vi "Teleop.vi"(10 "Match Info":T2={"Autonomous Elapsed Seconds"=0.0, "TeleOp Elapsed Seconds"=0.0, "Disabled Elapsed Seconds"=0.0, "Visited Autonomous"=FALSE, "Visited TeleOp"=FALSE, "Visited Disabled"=FALSE, "Autonomous Settings"={"Autonomous Style"=enum."Independent", "VI Refnum"=refnum}}, 11 "Call Context":T3=enum."Execute") -> ()   [LabVIEW 2018]
doc: "This VI is called for each TeleOp packet received from the DS where the robot is not disabled. It is often used to read from the joysticks and update I/O or to update setpoints for timed control loops. It should complete and return within 20 milliseconds or it may miss DS packets."
uses:
  <vilib>/Rock Robotics/WPI/DriverStation/WPI_DriverStationDerivedRobotMode.ctl
  <vilib>/Rock Robotics/WPI/DriverStation/WPI_DriverStationMatch Info.ctl
  <vilib>/Rock Robotics/WPI/Utilities/WPI_GetSetVariantRefNum.vi
  <vilib>/Rock Robotics/Network Tables/NT Write Boolean Array.vi
  <vilib>/Rock Robotics/Network Tables/NT Write Numeric Array.vi
  <vilib>/Rock Robotics/Network Tables/NT Read Boolean.vi
  <vilib>/Rock Robotics/Network Tables/NT Read Number.vi
  <vilib>/Rock Robotics/WPI/RobotDrive/WPI_RobotDriveArcadeDrive_Standard(NoSaturation).vi
  Robot Global Data.vi
  <vilib>/addons/control/pid/NI_PID_pid.lvlib
  <vilib>/Rock Robotics/WPI/ThirdParty/Phoenix-LabVIEW/Motor Controller/Controls/CTRE_Phoenix_MotorControl_ControlMode.ctl
  <vilib>/addons/control/pid/pid.llb/PID (DBL).vi
  <vilib>/Rock Robotics/WPI/ThirdParty/Phoenix-LabVIEW/Motor Controller/Get/CTRE_Phoenix_MotorController_GetQuadratureData.vi
  <vilib>/Rock Robotics/Network Tables/NT Write Boolean.vi
panel:
  in  "Sync PID":T1={"proportional gain (Kc)"=1.0, "integral time (Ti, min)"=0.01, "derivative time (Td, min)"=0.0} {"derivative time (Td, min)" format="%.3f"; "integral time (Ti, min)" format="%.3f"; "proportional gain (Kc)" format="%.3f"}
  in  "Drive PID":T1={"proportional gain (Kc)"=1.0, "integral time (Ti, min)"=0.01, "derivative time (Td, min)"=0.0} {"derivative time (Td, min)" format="%.3f"; "integral time (Ti, min)" format="%.3f"; "proportional gain (Kc)" format="%.3f"}
  in  "Mode":string(combo)="Driving"
  out "Drive Type":bool
  out "Sample Slider 0":dbl(slide) scale=0.0..5.0
  out "Sample Boolean 1":bool
  out "Sample Boolean 0":bool
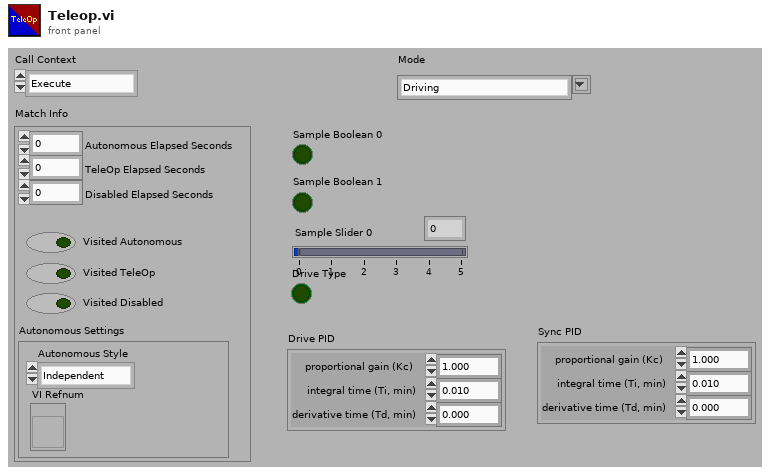
[diagram p1: front panel]
types:
  T1 = cluster{"proportional gain (Kc)":dbl, "integral time (Ti, min)":dbl, "derivative time (Td, min)":dbl}
  T2 = typedef "WPI_DriverStationMatch Info.ctl" = cluster{"Autonomous Elapsed Seconds":dbl, "TeleOp Elapsed Seconds":dbl, "Disabled Elapsed Seconds":dbl, "Visited Autonomous":bool, "Visited TeleOp":bool, "Visited Disabled":bool, "Autonomous Settings":cluster{"Autonomous Style":enum16{"Iterative", "Independent"}, "VI Refnum":refnum<vi>}}
  T3 = typedef "WPI_DriverStationDerivedRobotMode.ctl" = enum16{"Init", "Execute", "Stop"}
  T4 = typedef "WPI_JoystickDevRef.ctl" = cluster{"Device":T5}
  T5 = typedef "WPI_JoystickDeviceEnum.ctl" = enum16{"USB 0", "USB 1", "USB 2", "USB 3", "USB 4", "USB 5"}
  T6 = typedef "CTRE_Phoenix_MotorControl_ControlMode.ctl" = u16
  T7 = cluster{"Yaw":dbl, "Roll":dbl, "Pitch":dbl, "Heading":dbl, "Fused Heading":dbl}
  T8 = typedef "WPI_MotorControlDeviceRef.ctl" = cluster{"DeviceStatus":errorcluster, "Type":T9, "PWM":cluster{"PWM Channel":T10, "DeadBand":T11}, "CAN":cluster{"Device Number":u8, "SetOutput VI Ref":variant, "GetOutput VI Ref":variant, "Enable VI Ref":variant, "Disable VI Ref":variant, "Data":variant}, "Invert":bool, "DIO PWM":cluster{"PWM \"Enable\" Channel":T10, "DIOChannel":T12, "PWM Rate":dbl}}
  T9 = typedef "WPI_MotorControlType.ctl" = enum16{"PWM", "CAN", "DIO PWM"}
  T10 = typedef "FPGA_DIOPWMChannel.ctl" = enum8{"PWM 0", "PWM 1", "PWM 2", "PWM 3", "PWM 4", "PWM 5", "PWM 6", "PWM 7", "PWM 8", "PWM 9", "PWM MXP 0", "PWM MXP 1", "PWM MXP 2", "PWM MXP 3", "PWM MXP 4", "PWM MXP 5", "PWM MXP 6", "PWM MXP 7", "PWM MXP 8", "PWM MXP 9", "Invalid"}
  T11 = typedef "WPI_PWMDeadband.ctl" = cluster{"Name":string, "maxPositivePwm":i32, "minPositivePwm":i32, "centerPwm":i32, "maxNegativePwm":i32, "minNegativePwm":i32, "angularRange":u16}
  T12 = typedef "FPGA_DIOChannel.ctl" = enum8{"DIO 0", "DIO 1", "DIO 2", "DIO 3", "DIO 4", "DIO 5", "DIO 6", "DIO 7", "DIO 8", "DIO 9", "DIO MXP 0", "DIO MXP 1", "DIO MXP 2", "DIO MXP 3", "DIO MXP 4", "DIO MXP 5", "DIO MXP 6", "DIO MXP 7", "DIO MXP 8", "DIO MXP 9", "DIO MXP 10", "DIO MXP 11", "DIO MXP 12", "DIO MXP 13", "DIO MXP 14", "DIO MXP 15", "SPI Port CS1", "SPI Port CS2", "SPI Port CS3", "SPI Port MISO", "SPI Port MOSI", "Invalid"}
  T13 = typedef "WPI_RobotDriveDevRef.ctl" = cluster{"DevStatus":errorcluster, "Motors[]":T8[], "Square Inputs":bool, "Max Output":dbl}
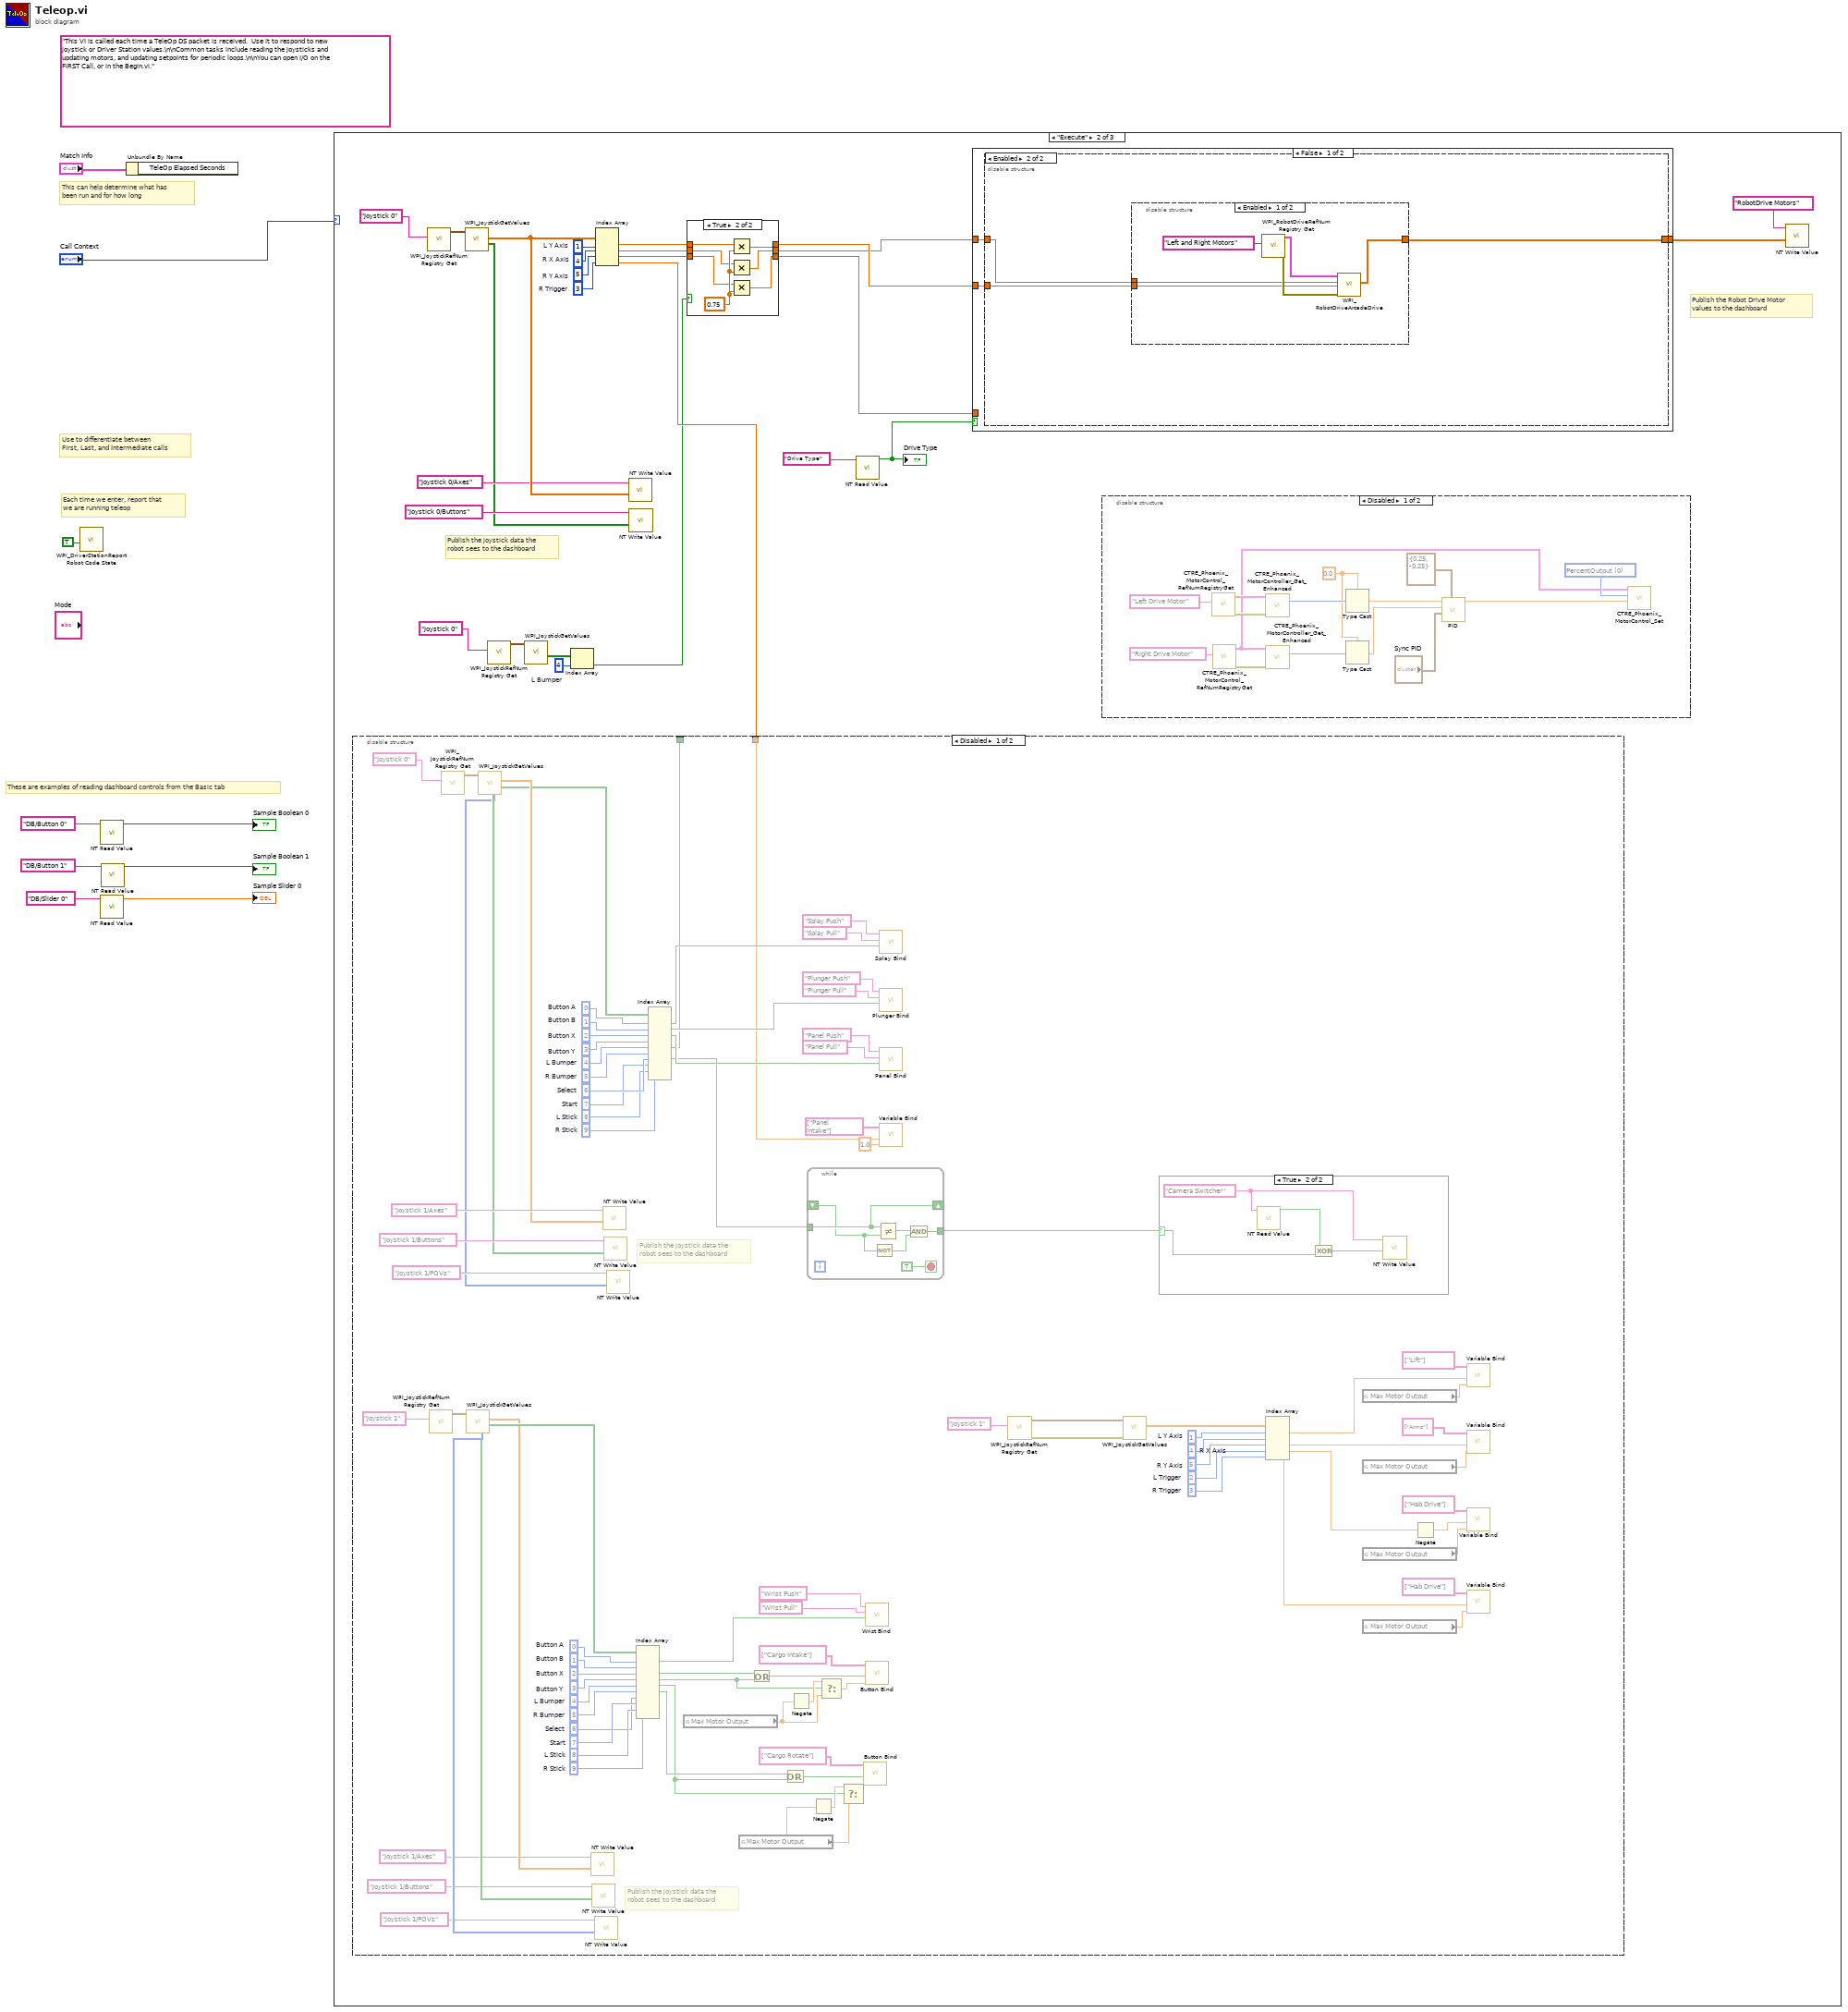
[diagram p0: block diagram]
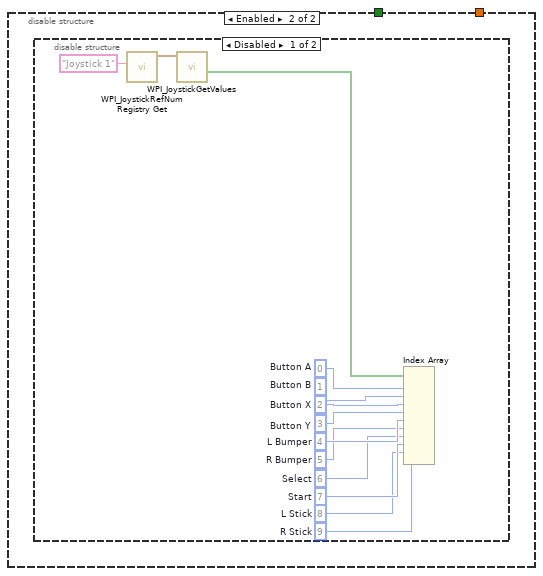
[diagram p4: hidden frame]
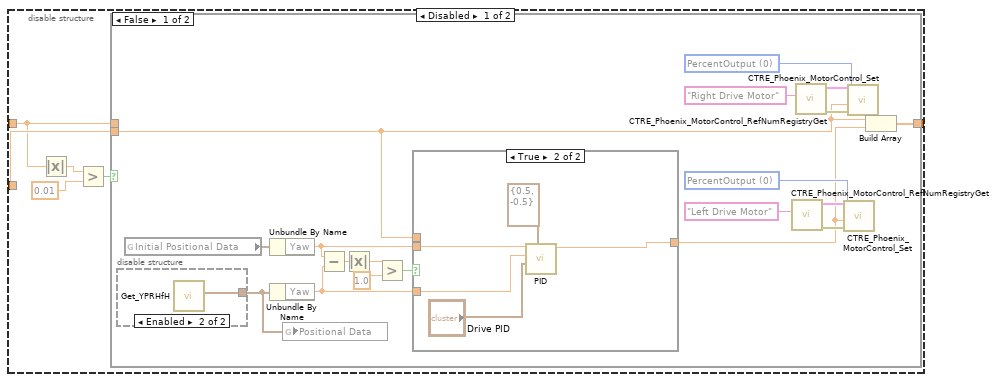
[diagram p7: hidden frame]
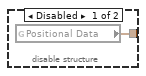
[diagram p8: hidden frame]
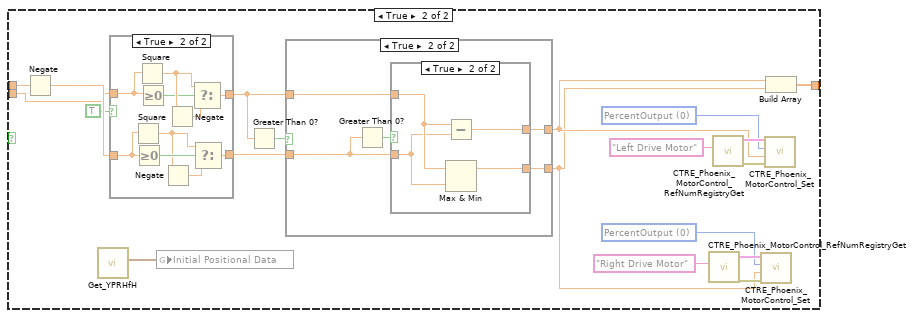
[diagram p10: hidden frame]
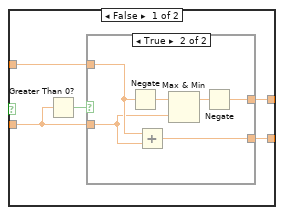
[diagram p11: hidden frame]
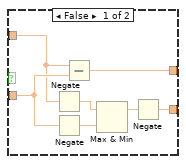
[diagram p12: hidden frame]
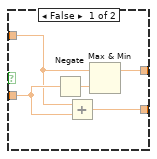
[diagram p13: hidden frame]
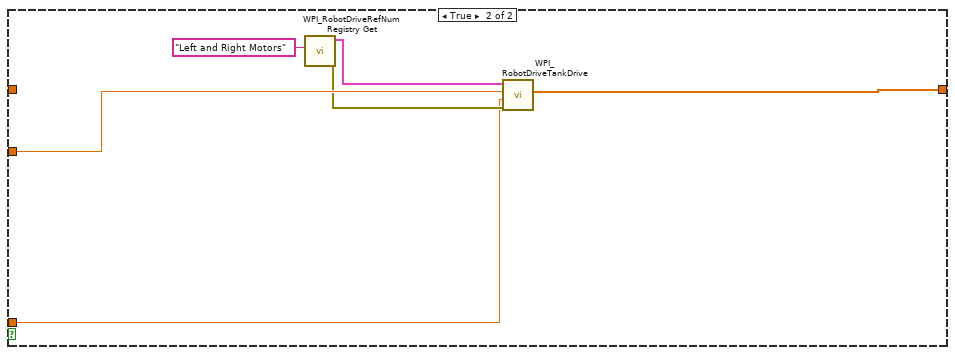
[diagram p16: hidden frame]
diagram:
  (unwired) "This VI is called each time a TeleOp DS packet is received.  Use it to respond to new joystick or Driver Station values.\n\nCommon tasks include reading the joysticks and updating motors, and updating setpoints for periodic loops.\n\nYou can open I/O on the FIRST Call, or in the Begin.vi."
  # "These are examples of reading dashboard controls from the Basic tab"
  # "Each time we enter, report that\nwe are running teleop"
  # "Use to differentiate between\nFirst, Last, and Intermediate calls"
  # "This can help determine what has\nbeen run and for how long"
  n1 = call <vilib>:"WPI_DriverStationReport Robot Code State.vi"("TeleOp"=TRUE ("Autonomous")) -> ()  [unwired: 10 in, 1 out]
  n2 = call-poly <vilib>:"NT Read Value.vi"("Name"="DB/Button 0" ("refnum name")) -> ("Boolean"=→"Sample Boolean 0":bool)  [unwired: 9 in, 1 out]
  n3 = call-poly <vilib>:"NT Read Value.vi"("Name"="DB/Slider 0" ("refnum name")) -> ("Numeric"=→"Sample Slider 0":dbl)  [unwired: 9 in, 1 out]
  n4 = call-poly <vilib>:"NT Read Value.vi"("Name"="DB/Button 1" ("refnum name")) -> ("Boolean"=→"Sample Boolean 1":bool)  [unwired: 9 in, 1 out]
  n5 = Unbundle By Name("Match Info") -> ()  [unwired: 1 out]
  n6 = case shown="\"Execute\"" "Call Context" {
    frame "Init", Default {
    }
    frame "Execute" {
      w12 = 4  # L Bumper
      w17 = 3  # R Trigger
      w28 = 4  # R X Axis
      w29 = 1  # L Y Axis
      w27 = 5  # R Y Axis
      # "Publish the Robot Drive Motor\nvalues to the dashboard"
      # "Publish the joystick data the\nrobot sees to the dashboard"
      n7 = call <vilib>:"WPI_JoystickRefNum Registry Get.vi"("refnum name"="Joystick 0") -> ("JoystickDevRef"=w34:T4)  [unwired: 1 in, 9 out]
      n8 = call <vilib>:"WPI_JoystickGetValues.vi"("JoystickDevRef"=w34) -> ("Buttons"=w26:bool[], "Axes"=w35:dbl[])  [unwired: 6 in, 3 out]
      n9 = call <vilib>:"WPI_JoystickRefNum Registry Get.vi"("refnum name"="Joystick 0") -> ("JoystickDevRef"=w14:T4)  [unwired: 1 in, 9 out]
      n10 = call <vilib>:"WPI_JoystickGetValues.vi"("JoystickDevRef"=w14) -> ("Buttons"=w10:bool[])  [unwired: 6 in, 4 out]
      n11 = Index Array(array=w10, index=w12) -> (element=w11:bool)
      n12 = Index Array(array=w35, index #1=w29, index #2=w28, index #3=w27, index #4=w17) -> (element #1=w25:dbl, element #2=w22:dbl, element #3=w21:dbl, element #4=w16:dbl)
      n13 = disable-structure shown="Disabled" {
        disable-tunnel: [w102 _] -> _
        disable-tunnel: w16 -> [w44 _]
        frame Disabled {
          w60 = 3  # R Trigger
          w61 = 2  # L Trigger
          w63 = 4  # R X Axis
          w64 = 1  # L Y Axis
          w62 = 5  # R Y Axis
          w99 = 9  # R Stick
          w98 = 8  # L Stick
          w97 = 7  # Start
          w96 = 6  # Select
          w95 = 5  # R Bumper
          w94 = 4  # L Bumper
          w82 = 3  # Button Y
          w85 = 1  # Button B
          w83 = 0  # Button A
          w84 = 2  # Button X
          w104 = 9  # R Stick
          w105 = 8  # L Stick
          w106 = 7  # Start
          w107 = 6  # Select
          w112 = 5  # R Bumper
          w113 = 4  # L Bumper
          w125 = 3  # Button Y
          w122 = 1  # Button B
          w124 = 0  # Button A
          w123 = 2  # Button X
          # "Publish the joystick data the\nrobot sees to the dashboard"
          # "Publish the joystick data the\nrobot sees to the dashboard"
          n14 = call <vilib>:"WPI_JoystickRefNum Registry Get.vi"("refnum name"="Joystick 1") -> ("JoystickDevRef"=w87:T4)  [unwired: 1 in, 9 out]
          n15 = call <vilib>:"WPI_JoystickRefNum Registry Get.vi"("refnum name"="Joystick 0") -> ("JoystickDevRef"=w120:T4)  [unwired: 1 in, 9 out]
          n16 = call <vilib>:"WPI_JoystickGetValues.vi"("JoystickDevRef"=w87) -> ("Buttons"=w91:bool[], "Axes"=w90:dbl[], "POVs"=w93:i16[])  [unwired: 6 in, 2 out]
          n17 = call <vilib>:"WPI_JoystickGetValues.vi"("JoystickDevRef"=w120) -> ("Buttons"=w116:bool[], "Axes"=w117:dbl[], "POVs"=w114:i16[])  [unwired: 6 in, 2 out]
          n18 = call-poly <vilib>:"NT Write Value.vi"("Numeric Array"=w90, "Name"="Joystick 1/Axes") -> ()  [unwired: 9 in, 1 out]
          n19 = call-poly <vilib>:"NT Write Value.vi"("Boolean Array"=w91, "Name"="Joystick 1/Buttons") -> ()  [unwired: 9 in, 1 out]
          n20 = call-poly <vilib>:"NT Write Value.vi"("Numeric Array"=w93, "Name"="Joystick 1/POVs") -> ()  [unwired: 9 in, 1 out]
          n21 = call-poly <vilib>:"NT Write Value.vi"("Numeric Array"=w117, "Name"="Joystick 1/Axes") -> ()  [unwired: 9 in, 1 out]
          n22 = call-poly <vilib>:"NT Write Value.vi"("Boolean Array"=w116, "Name"="Joystick 1/Buttons") -> ()  [unwired: 9 in, 1 out]
          n23 = call-poly <vilib>:"NT Write Value.vi"("Numeric Array"=w114, "Name"="Joystick 1/POVs") -> ()  [unwired: 9 in, 1 out]
          n24 = Index Array(array=w91, index #1=w83, index #2=w85, index #3=w84, index #4=w82, index #5=w94, index #6=w95, index #7=w96, index #8=w97, index #9=w98, index #10=w99) -> (element #1=w77:bool, element #3=w40:bool, element #4=w37:bool, element #5=w36:bool, element #6=w81:bool)  [unwired: 5 out]
          n25 = Index Array(array=w116, index #1=w124, index #2=w122, index #3=w123, index #4=w125, index #5=w113, index #6=w112, index #7=w107, index #8=w106, index #9=w105, index #10=w104) -> (element #1=w108:bool, element #2=w111:bool, element #3=w103:bool, element #5=w102:bool, element #7=w46:bool)  [unwired: 5 out]
          n26 = global read "Robot Global Data.vi" "Max Motor Output"() -> (w41:dbl)
          n27 = global read "Robot Global Data.vi" "Max Motor Output"() -> (w73:dbl)
          n28 = Or(x=w40, y=w37) -> (x .or. y?=w38:bool)
          n29 = Or(x=w81, y=w36) -> (x .or. y?=w76:bool)
          n30 = Negate(x=w41) -> (-x=w42:dbl)
          n31 = while {
            shift-right: [w135] -> _
            shift-left: _ -> [w133]
            tunnel: w46 -> [w135]
            tunnel: [w132] -> w45
            stop <- TRUE stop-if-true
            n32 = Not(x=w133) -> (.not. x?=w130:bool)
            n33 = Not Equal?(x=w135, y=w133) -> (x != y?=w131:bool)
            n34 = And(x=w131, y=w130) -> (x .and. y?=w132:bool)
          }
          n35 = Negate(x=w73) -> (-x=w74:dbl)
          n36 = Select(t=w42, s=w37, f=w41) -> (s? t:f=w39:dbl)
          n37 = Select(t=w74, s=w36, f=w73) -> (s? t:f=w75:dbl)
          n38 = call "Button Bind.vi"("Output"=w75, "Button ID"=w76, "PhoenixMotorControlDevRef"=string[] ["Cargo Rotate"] ("Motor Controllers")) -> ()  [unwired: 8 in, 1 out]
          n39 = call "Wrist Bind.vi"("Button Input"=w77, "Pull Solenoid Ref"="Wrist Pull" ("Push Solenoid Ref"), "Push Solenoid Ref"="Wrist Push") -> ()  [unwired: 9 in]
          n40 = call "Button Bind.vi"("Output"=w39, "Button ID"=w38, "PhoenixMotorControlDevRef"=string[] ["Cargo Intake"] ("Motor Controllers")) -> ()  [unwired: 8 in, 1 out]
          n41 = call "Splay Bind.vi"("Button Input"=w108, "Pull Solenoid Ref"="Splay Pull" ("Push Solenoid Ref"), "Push Solenoid Ref"="Splay Push") -> ()  [unwired: 9 in]
          n42 = call "Plunger Bind.vi"("Button Input"=w111, "Pull Solenoid Ref"="Plunger Pull" ("Push Solenoid Ref"), "Push Solenoid Ref"="Plunger Push") -> ()  [unwired: 9 in]
          n43 = call "Panel Bind.vi"("Button Input"=w103, "Pull Solenoid Ref"="Panel Pull" ("Push Solenoid Ref"), "Push Solenoid Ref"="Panel Push") -> ()  [unwired: 9 in]
          n44 = call "Variable Bind.vi"("Ouput"=1.0 ("Max Ouput"), "Axis ID"=w44, "PhoenixMotorControlDevRef"=string[] ["Panel Intake"] ("Motor Controllers")) -> ()  [unwired: 8 in, 1 out]
          n45 = call <vilib>:"WPI_JoystickRefNum Registry Get.vi"("refnum name"="Joystick 1") -> ("error out"=w66:errorcluster, "JoystickDevRef"=w67:T4)  [unwired: 1 in, 8 out]
          n46 = call <vilib>:"WPI_JoystickGetValues.vi"("error in (no error)"=w66, "JoystickDevRef"=w67) -> ("Axes"=w65:dbl[])  [unwired: 5 in, 4 out]
          n47 = case shown="True" w45 {
            selector: w45 -> [_ w129]
            frame False {
            }
            frame True {
              w127 = "Camera Switcher" ("Name")
              n48 = call-poly <vilib>:"NT Read Value.vi"("Name"=w127) -> ("Boolean"=w126:bool)  [unwired: 9 in, 1 out]
              n49 = Exclusive Or(1:w129, 2:w126) -> (0:w128:bool)
              n50 = call-poly <vilib>:"NT Write Value.vi"("Boolean"=w128, "Name"=w127) -> ()  [unwired: 9 in, 1 out]
            }
          }
          n51 = Index Array(array=w65, index #1=w64, index #2=w63, index #3=w62, index #4=w61, index #5=w60) -> (element #1=w50:dbl, element #3=w49:dbl, element #4=w58:dbl, element #5=w53:dbl)  [unwired: 1 out]
          n52 = global read "Robot Global Data.vi" "Max Motor Output"() -> (w51:dbl)
          n53 = global read "Robot Global Data.vi" "Max Motor Output"() -> (w47:dbl)
          n54 = global read "Robot Global Data.vi" "Max Motor Output"() -> (w56:dbl)
          n55 = global read "Robot Global Data.vi" "Max Motor Output"() -> (w55:dbl)
          n56 = Negate(x=w58) -> (-x=w57:dbl)
          n57 = call "Variable Bind.vi"("Ouput"=w51, "Axis ID"=w50, "PhoenixMotorControlDevRef"=string[] ["Lift"] ("Motor Controllers")) -> ()  [unwired: 8 in, 1 out]
          n58 = call "Variable Bind.vi"("Ouput"=w47, "Axis ID"=w49, "PhoenixMotorControlDevRef"=string[] ["Arms"] ("Motor Controllers")) -> ()  [unwired: 8 in, 1 out]
          n59 = call "Variable Bind.vi"("Ouput"=w56, "Axis ID"=w57, "PhoenixMotorControlDevRef"=string[] ["Hab Drive"] ("Motor Controllers")) -> ()  [unwired: 8 in, 1 out]
          n60 = call "Variable Bind.vi"("Ouput"=w55, "Axis ID"=w53, "PhoenixMotorControlDevRef"=string[] ["Hab Drive"] ("Motor Controllers")) -> ()  [unwired: 8 in, 1 out]
        }
        frame Enabled {
          n61 = disable-structure shown="Disabled" {
            frame Disabled {
              w138 = 9  # R Stick
              w139 = 8  # L Stick
              w140 = 7  # Start
              w141 = 6  # Select
              w142 = 5  # R Bumper
              w143 = 4  # L Bumper
              w144 = 3  # Button Y
              w146 = 1  # Button B
              w147 = 0  # Button A
              w145 = 2  # Button X
              n62 = call <vilib>:"WPI_JoystickRefNum Registry Get.vi"("refnum name"="Joystick 1") -> ("JoystickDevRef"=w148:T4)  [unwired: 1 in, 9 out]
              n63 = call <vilib>:"WPI_JoystickGetValues.vi"("JoystickDevRef"=w148) -> ("Buttons"=w137:bool[])  [unwired: 6 in, 4 out]
              n64 = Index Array(array=w137, index #1=w147, index #2=w146, index #3=w145, index #4=w144, index #5=w143, index #6=w142, index #7=w141, index #8=w140, index #9=w139, index #10=w138) -> ()  [unwired: 10 out]
            }
            frame Enabled {
            }
          }
        }
      }
      n65 = call-poly <vilib>:"NT Write Value.vi"("Numeric Array"=w35, "Name"="Joystick 0/Axes") -> ()  [unwired: 9 in, 1 out]
      n66 = call-poly <vilib>:"NT Write Value.vi"("Boolean Array"=w26, "Name"="Joystick 0/Buttons") -> ()  [unwired: 9 in, 1 out]
      n67 = case shown="True" w11 {
        tunnel: w25 -> [w280 w286]
        tunnel: [w280 w285] -> w24
        tunnel: [w279 w283] -> w23
        tunnel: w22 -> [w279 w284]
        tunnel: [w278 w281] -> w20
        tunnel: w21 -> [w278 w282]
        frame False {
        }
        frame True {
          w287 = 0.75 ("y")
          n68 = Multiply(x=w286, y=w287) -> (x*y=w285:dbl)
          n69 = Multiply(x=w284, y=w287) -> (x*y=w283:dbl)
          n70 = Multiply(x=w282, y=w287) -> (x*y=w281:dbl)
        }
      }
      n71 = call-poly <vilib>:"NT Read Value.vi"("Name"="Drive Type" ("refnum name")) -> ("Boolean"=w18:bool)  [unwired: 9 in, 1 out]
      "Drive Type" <- w18
      n72 = case shown="False" w18 {
        tunnel: w20 -> [_ w272]
        tunnel: w23 -> [w165 _]
        tunnel: w24 -> [w166 w277]
        tunnel: [w164 w273] -> w15
        frame False {
          n73 = disable-structure shown="Enabled" {
            disable-tunnel: w166 -> [w172 w264]
            disable-tunnel: w165 -> [w167 w265]
            disable-tunnel: [w168 w263] -> w164
            frame Disabled {
              n74 = Absolute Value(x=w167) -> (abs(x)=w170:dbl)
              n75 = Greater?(x=w170, y=0.01) -> (0:w169:bool)
              n76 = case shown="False" w169 {
                tunnel: [w182 w211] -> w168
                tunnel: w172 -> [w176 w213]
                tunnel: w167 -> [_ w218]
                frame False {
                  w187 = T6 0 items=["PercentOutput"=0, "Position"=1, "Velocity"=2, "Current"=3, "Follower"=5, "MotionProfile"=6, "MotionMagic"=7, "MotionProfileArc"=10, "Disabled"=15] ("Control Mode")
                  w188 = T6 0 items=["PercentOutput"=0, "Position"=1, "Velocity"=2, "Current"=3, "Follower"=5, "MotionProfile"=6, "MotionMagic"=7, "MotionProfileArc"=10, "Disabled"=15] ("Control Mode")
                  n77 = disable-structure shown="Enabled" {
                    disable-tunnel: [w192 w193] -> w173
                    frame Disabled {
                      n78 = global read "Robot Global Data.vi" "Positional Data"() -> (w192:T7)
                    }
                    frame Enabled {
                      n79 = call <vilib>:"Get_YPRHfH.vi"() -> ("YRPHfH"=w193:T7)  [unwired: 11 in]
                    }
                  }
                  n80 = global read "Robot Global Data.vi" "Initial Positional Data"() -> (w181:T7)
                  n81 = Unbundle By Name(w181) -> ("Yaw"=w179:dbl)
                  n82 = Unbundle By Name(w173) -> ("Yaw"=w175:dbl)
                  n83 = global write "Robot Global Data.vi" "Positional Data"(w173) -> ()
                  n84 = Subtract(x=w179, y=w175) -> (x-y=w180:dbl)
                  n85 = Absolute Value(x=w180) -> (abs(x)=w177:dbl)
                  n86 = Greater?(x=w177, y=1.0) -> (0:w174:bool)
                  n87 = case shown="True" w174 {
                    tunnel: w175 -> [_ w199]
                    tunnel: [w194 w196] -> w183
                    tunnel: w176 -> [w194 _]
                    tunnel: w179 -> [_ w197]
                    frame False {
                    }
                    frame True {
                      n88 = call-poly <vilib>:"PID.vi"("output range"=cluster{"output high":dbl, "output low":dbl} {"output high"=0.5, "output low"=-0.5}, "PID gains"="Drive PID", "process variable"=w199, "setpoint"=w197) -> ("output"=w196:dbl)  [unwired: 6 in, 1 out]
                    }
                  }
                  n89 = call <vilib>:"CTRE_Phoenix_MotorControl_RefNumRegistryGet.vi"("refnum name"="Left Drive Motor") -> ("error out"=w185:errorcluster, "PhoenixMotorControlDevRef"=w186:T8)  [unwired: 9 in]
                  n90 = call <vilib>:"CTRE_Phoenix_MotorControl_RefNumRegistryGet.vi"("refnum name"="Right Drive Motor") -> ("error out"=w190:errorcluster, "PhoenixMotorControlDevRef"=w189:T8)  [unwired: 9 in]
                  n91 = call <vilib>:"CTRE_Phoenix_MotorControl_Set.vi"("error in (no error)"=w185, "Output"=w183, "Control Mode"=w187, "PhoenixMotorControlDevRef"=w186) -> ()  [unwired: 6 in, 2 out]
                  n92 = call <vilib>:"CTRE_Phoenix_MotorControl_Set.vi"("error in (no error)"=w190, "Output"=w176, "Control Mode"=w188, "PhoenixMotorControlDevRef"=w189) -> ()  [unwired: 6 in, 2 out]
                  n93 = Build Array(w176, w183) -> (w182:dbl[])
                }
                frame True {
                  w206 = T6 0 items=["PercentOutput"=0, "Position"=1, "Velocity"=2, "Current"=3, "Follower"=5, "MotionProfile"=6, "MotionMagic"=7, "MotionProfileArc"=10, "Disabled"=15] ("Control Mode")
                  w204 = T6 0 items=["PercentOutput"=0, "Position"=1, "Velocity"=2, "Current"=3, "Follower"=5, "MotionProfile"=6, "MotionMagic"=7, "MotionProfileArc"=10, "Disabled"=15] ("Control Mode")
                  n94 = Negate(x=w218) -> (-x=w214:dbl)
                  n95 = call <vilib>:"Get_YPRHfH.vi"() -> ("YRPHfH"=w200:T7)  [unwired: 11 in]
                  n96 = case shown="True" TRUE {
                    tunnel: [w251 w262] -> w215
                    tunnel: [w252 w261] -> w216
                    tunnel: w214 -> [w251 w260]
                    tunnel: w213 -> [w252 w259]
                    frame False {
                    }
                    frame True {
                      n97 = Square(x=w260) -> (x^2=w257:dbl)
                      n98 = Greater Or Equal To 0?(x=w260) -> (x >= 0?=w258:bool)
                      n99 = Square(x=w259) -> (x^2=w254:dbl)
                      n100 = Greater Or Equal To 0?(x=w259) -> (x >= 0?=w253:bool)
                      n101 = Negate(x=w257) -> (-x=w256:dbl)
                      n102 = Negate(x=w254) -> (-x=w255:dbl)
                      n103 = Select(t=w254, s=w253, f=w255) -> (s? t:f=w261:dbl)
                      n104 = Select(t=w257, s=w258, f=w256) -> (s? t:f=w262:dbl)
                    }
                  }
                  n105 = global write "Robot Global Data.vi" "Initial Positional Data"(w200) -> ()
                  n106 = Greater Than 0?(x=w216) -> (x > 0?=w217:bool)
                  n107 = case shown="True" w217 {
                    tunnel: w215 -> [w222 w240]
                    tunnel: w216 -> [w221 w239]
                    tunnel: [w220 w238] -> w202
                    tunnel: [w219 w237] -> w201
                    frame False {
                      n108 = Greater Than 0?(x=w222) -> (x > 0?=w223:bool)
                      n109 = case shown="True" w223 {
                        tunnel: w222 -> [w230 w232]
                        tunnel: w221 -> [w228 w233]
                        tunnel: [w224 w234] -> w220
                        tunnel: [w225 w231] -> w219
                        frame False {
                          n110 = Negate(x=w228) -> (-x=w229:dbl)
                          n111 = Negate(x=w230) -> (-x=w227:dbl)
                          n112 = Subtract(x=w228, y=w230) -> (x-y=w224:dbl)
                          n113 = Max & Min(x=w229, y=w227) -> (max(x,y)=w226:dbl)  [unwired: 1 out]
                          n114 = Negate(x=w226) -> (-x=w225:dbl)
                        }
                        frame True {
                          n115 = Negate(x=w233) -> (-x=w236:dbl)
                          n116 = Add(x=w233, y=w232) -> (x+y=w231:dbl)
                          n117 = Max & Min(x=w236, y=w232) -> (max(x,y)=w235:dbl)  [unwired: 1 out]
                          n118 = Negate(x=w235) -> (-x=w234:dbl)
                        }
                      }
                    }
                    frame True {
                      n119 = Greater Than 0?(x=w240) -> (x > 0?=w241:bool)
                      n120 = case shown="True" w241 {
                        tunnel: w240 -> [w246 w248]
                        tunnel: w239 -> [w243 w249]
                        tunnel: [w244 w247] -> w238
                        tunnel: [w242 w250] -> w237
                        frame False {
                          n121 = Negate(x=w246) -> (-x=w245:dbl)
                          n122 = Add(x=w243, y=w246) -> (x+y=w242:dbl)
                          n123 = Max & Min(x=w243, y=w245) -> (max(x,y)=w244:dbl)  [unwired: 1 out]
                        }
                        frame True {
                          n124 = Subtract(x=w249, y=w248) -> (x-y=w247:dbl)
                          n125 = Max & Min(x=w249, y=w248) -> (max(x,y)=w250:dbl)  [unwired: 1 out]
                        }
                      }
                    }
                  }
                  n126 = call <vilib>:"CTRE_Phoenix_MotorControl_RefNumRegistryGet.vi"("refnum name"="Right Drive Motor") -> ("error out"=w208:errorcluster, "PhoenixMotorControlDevRef"=w207:T8)  [unwired: 9 in]
                  n127 = call <vilib>:"CTRE_Phoenix_MotorControl_RefNumRegistryGet.vi"("refnum name"="Left Drive Motor") -> ("error out"=w209:errorcluster, "PhoenixMotorControlDevRef"=w210:T8)  [unwired: 9 in]
                  n128 = call <vilib>:"CTRE_Phoenix_MotorControl_Set.vi"("error in (no error)"=w208, "Output"=w201, "Control Mode"=w206, "PhoenixMotorControlDevRef"=w207) -> ()  [unwired: 6 in, 2 out]
                  n129 = call <vilib>:"CTRE_Phoenix_MotorControl_Set.vi"("error in (no error)"=w209, "Output"=w202, "Control Mode"=w204, "PhoenixMotorControlDevRef"=w210) -> ()  [unwired: 6 in, 2 out]
                  n130 = Build Array(w202, w201) -> (w211:dbl[])
                }
              }
            }
            frame Enabled {
              n131 = disable-structure shown="Enabled" {
                disable-tunnel: w265 -> [w268 _]
                disable-tunnel: w264 -> [w267 _]
                disable-tunnel: [w266 _] -> w263
                frame Enabled {
                  n132 = call <vilib>:"WPI_RobotDriveRefNum Registry Get.vi"("refnum name"="Left and Right Motors") -> ("error out"=w270:errorcluster, "RobotDriveDevRef"=w271:T13)  [unwired: 9 in]
                  n133 = call-poly <vilib>:"WPI_RobotDriveArcadeDrive.vi"("error in (no error)"=w270, "Y axis value"=w267, "X axis value"=w268, "RobotDriveDevRef"=w271) -> ("Motor Values"=w266:dbl[])  [unwired: 5 in, 2 out]
                }
                frame Disabled {
                }
              }
            }
          }
        }
        frame True {
          n134 = call <vilib>:"WPI_RobotDriveRefNum Registry Get.vi"("refnum name"="Left and Right Motors") -> ("error out"=w274:errorcluster, "RobotDriveDevRef"=w275:T13)  [unwired: 9 in]
          n135 = call <vilib>:"WPI_RobotDriveTankDrive.vi"("error in (no error)"=w274, "Right axis value"=w272, "Left axis value"=w277, "RobotDriveDevRef"=w275) -> ("Motor Values"=w273:dbl[])  [unwired: 5 in, 2 out]
        }
      }
      n136 = disable-structure shown="Disabled" {
        frame Disabled {
          w152 = T6 0 items=["PercentOutput"=0, "Position"=1, "Velocity"=2, "Current"=3, "Follower"=5, "MotionProfile"=6, "MotionMagic"=7, "MotionProfileArc"=10, "Disabled"=15] ("Control Mode")
          w154 = 0.0
          n137 = call <vilib>:"CTRE_Phoenix_MotorControl_RefNumRegistryGet.vi"("refnum name"="Left Drive Motor") -> ("error out"=w163:errorcluster, "PhoenixMotorControlDevRef"=w162:T8)  [unwired: 9 in]
          n138 = call <vilib>:"CTRE_Phoenix_MotorControl_RefNumRegistryGet.vi"("refnum name"="Right Drive Motor") -> ("error out"=w159:errorcluster, "PhoenixMotorControlDevRef"=w150:T8)  [unwired: 9 in]
          n139 = call-poly <vilib>:"CTRE_Phoenix_MotorController_Get_Enhanced.vi"("PhoenixMotorControlDevRef"=w162, "error in"=w163) -> ("Quadrature Position"=w157:i32)  [unwired: 10 in, 3 out]
          n140 = call-poly <vilib>:"CTRE_Phoenix_MotorController_Get_Enhanced.vi"("PhoenixMotorControlDevRef"=w150, "error in"=w159) -> ("Quadrature Position"=w155:i32)  [unwired: 10 in, 3 out]
          n141 = Type Cast(type=w154, x=w157) -> (*(type *) &x=w156:dbl)
          n142 = Type Cast(type=w154, x=w155) -> (*(type *) &x=w153:dbl)
          n143 = call-poly <vilib>:"PID.vi"("output range"=cluster{"output high":dbl, "output low":dbl} {"output high"=0.25, "output low"=-0.25}, "PID gains"="Sync PID", "process variable"=w153, "setpoint"=w156) -> ("output"=w151:dbl)  [unwired: 6 in, 1 out]
          n144 = call <vilib>:"CTRE_Phoenix_MotorControl_Set.vi"("Output"=w151, "Control Mode"=w152, "PhoenixMotorControlDevRef"=w150) -> ()  [unwired: 7 in, 2 out]
        }
        frame Enabled {
        }
      }
      n145 = call-poly <vilib>:"NT Write Value.vi"("Numeric Array"=w15, "Name"="RobotDrive Motors") -> ()  [unwired: 9 in, 1 out]
    }
    frame "Stop" {
    }
  }
